vi "Scan Module.vi"(7 "Slice pattern":T1={"repitition"=14, "thick slice (um)"=500.0, "thin slice (um)"=100.0} {"thin slice (um)" format="%#_13g"; "thick slice (um)" format="%#_13g"}, 8 "Error In":errorcluster, 9 "System Parameters":T2={"Vibratome"={"Z Bottom [mm]"=0.0, "Pre Cut Dwell [s]"=1.0, "Blade Frequency [RPM]"=3000, "Slice Speed [mm/s]"=0.1, "Post Cut Dwell [s]"=4.0, "Ramp Time [s]"=0.5, "Start X [mm]"=80.5, "Start Y [mm]"=72.0, "Slice Length [mm]"=15.0, "Slice Axis"=enum."X Axis", "Controller VISA Ref"="COM3"}, "Table Stages"={"X Stage"={"Position"=0.0, "Is.Enabled?"=FALSE, "Is.Connected?"=FALSE, "Device SN"="45875688", "AccelerationMaximum"=50.0, "VelocityMaximum"=50.0, "Acceleration"=20.0, "Velocity"=20.0, "waitTimeout (ms)"=1000000, "Model"=enum."Thorlabs LTS", "Is.Homed?"=FALSE}, "Y Stage"={"Position"=0.0, "Is.Enabled?"=FALSE, "Is.Connected?"=FALSE, "Device SN"="45875512", "AccelerationMaximum"=50.0, "VelocityMaximum"=50.0, "Acceleration"=20.0, "Velocity"=20.0, "waitTimeout (ms)"=1000000, "Model"=enum."Thorlabs LTS", "Is.Homed?"=FALSE}, "Z Stage"={"Position"=0.0, "Is.Enabled?"=FALSE, "Is.Connected?"=FALSE, "Device SN"="49872414", "AccelerationMaximum"=50.0, "VelocityMaximum"=50.0, "Acceleration"=20.0, "Velocity"=20.0, "waitTimeout (ms)"=100000, "Model"=enum."Thorlabs MLJ", "Is.Homed?"=FALSE}}}, 10 "Mosaic Parameters":T5={"Overlap Options"={"Overlap Type"=enum."No Overlap", "Percent Overlap"=0, "Justify"=enum."Start"}, "Mosaic Range"={"X Axis"={"Start [mm]"=10.0, "Steps [pts]"=0, "End [mm]"=28.0}, "Y Axis"={"Start [mm]"=45.0, "Steps [pts]"=0, "End [mm]"=63.0}}, "Scan Pattern"=enum."Uni-directional", "Number of slices"=1} {"Overlap Options"."Percent Overlap" max=50}, 11 "Imaging Parameters":T6={"Save Path"=path "E:/Jiarui/1217test", "# Cscan"=1, "ROI Parameters"={"ROI (mm)"={"X (mm)"=1.0, "Y (mm)"=1.0}, "Shift (mm)"={"Xshift (mm)"=0.0, "Yshift (mm)"=0.0}}, "Scan Parameters"={"# Scan"={"#Ascan"=400, "#Bscan"=400}, "# Rpt"={"#ARpt"=1, "#BRpt"=1}, "Aline Rate"=2, "# Extra"={"# ARpt_extra"=5, "#Brtn_extra"=80}}, "Objective"=0, "Image Index"=0} {"Objective" items=["5X LKM05", "10X LKM10", "20X LKM20", "10X LSM02"]; "Scan Parameters"."Aline Rate" items=["76 KHz", "146 KHz", "76 KHz", "28 KHz", "10 KHz"]}) -> (0 "Error Out":errorcluster, 3 "Finished?":bool)   [LabVIEW 2017]
uses:
  Controls/Go Scan Actions.ctl
  Controls/System Parameters.ctl
  Hardware/Table Stage/Controls/Translation Stage Cluster.ctl
  Controls/Translation Stage Types.ctl
  Controls/FGV Actions.ctl
  Controls/ScanType.ctl
  Hardware/Table Stage/Controls/Motion Translation Module Control.ctl
  Controls/Set Get Controls.ctl
panel:
  out "Waveform Chart":dbl(graph)
  out "Current State":T7
  out "Current Position":cluster{"X":dbl, "Y":dbl}
  out "XY Graph":cluster{"X":dbl, "Y":dbl}[](graph)
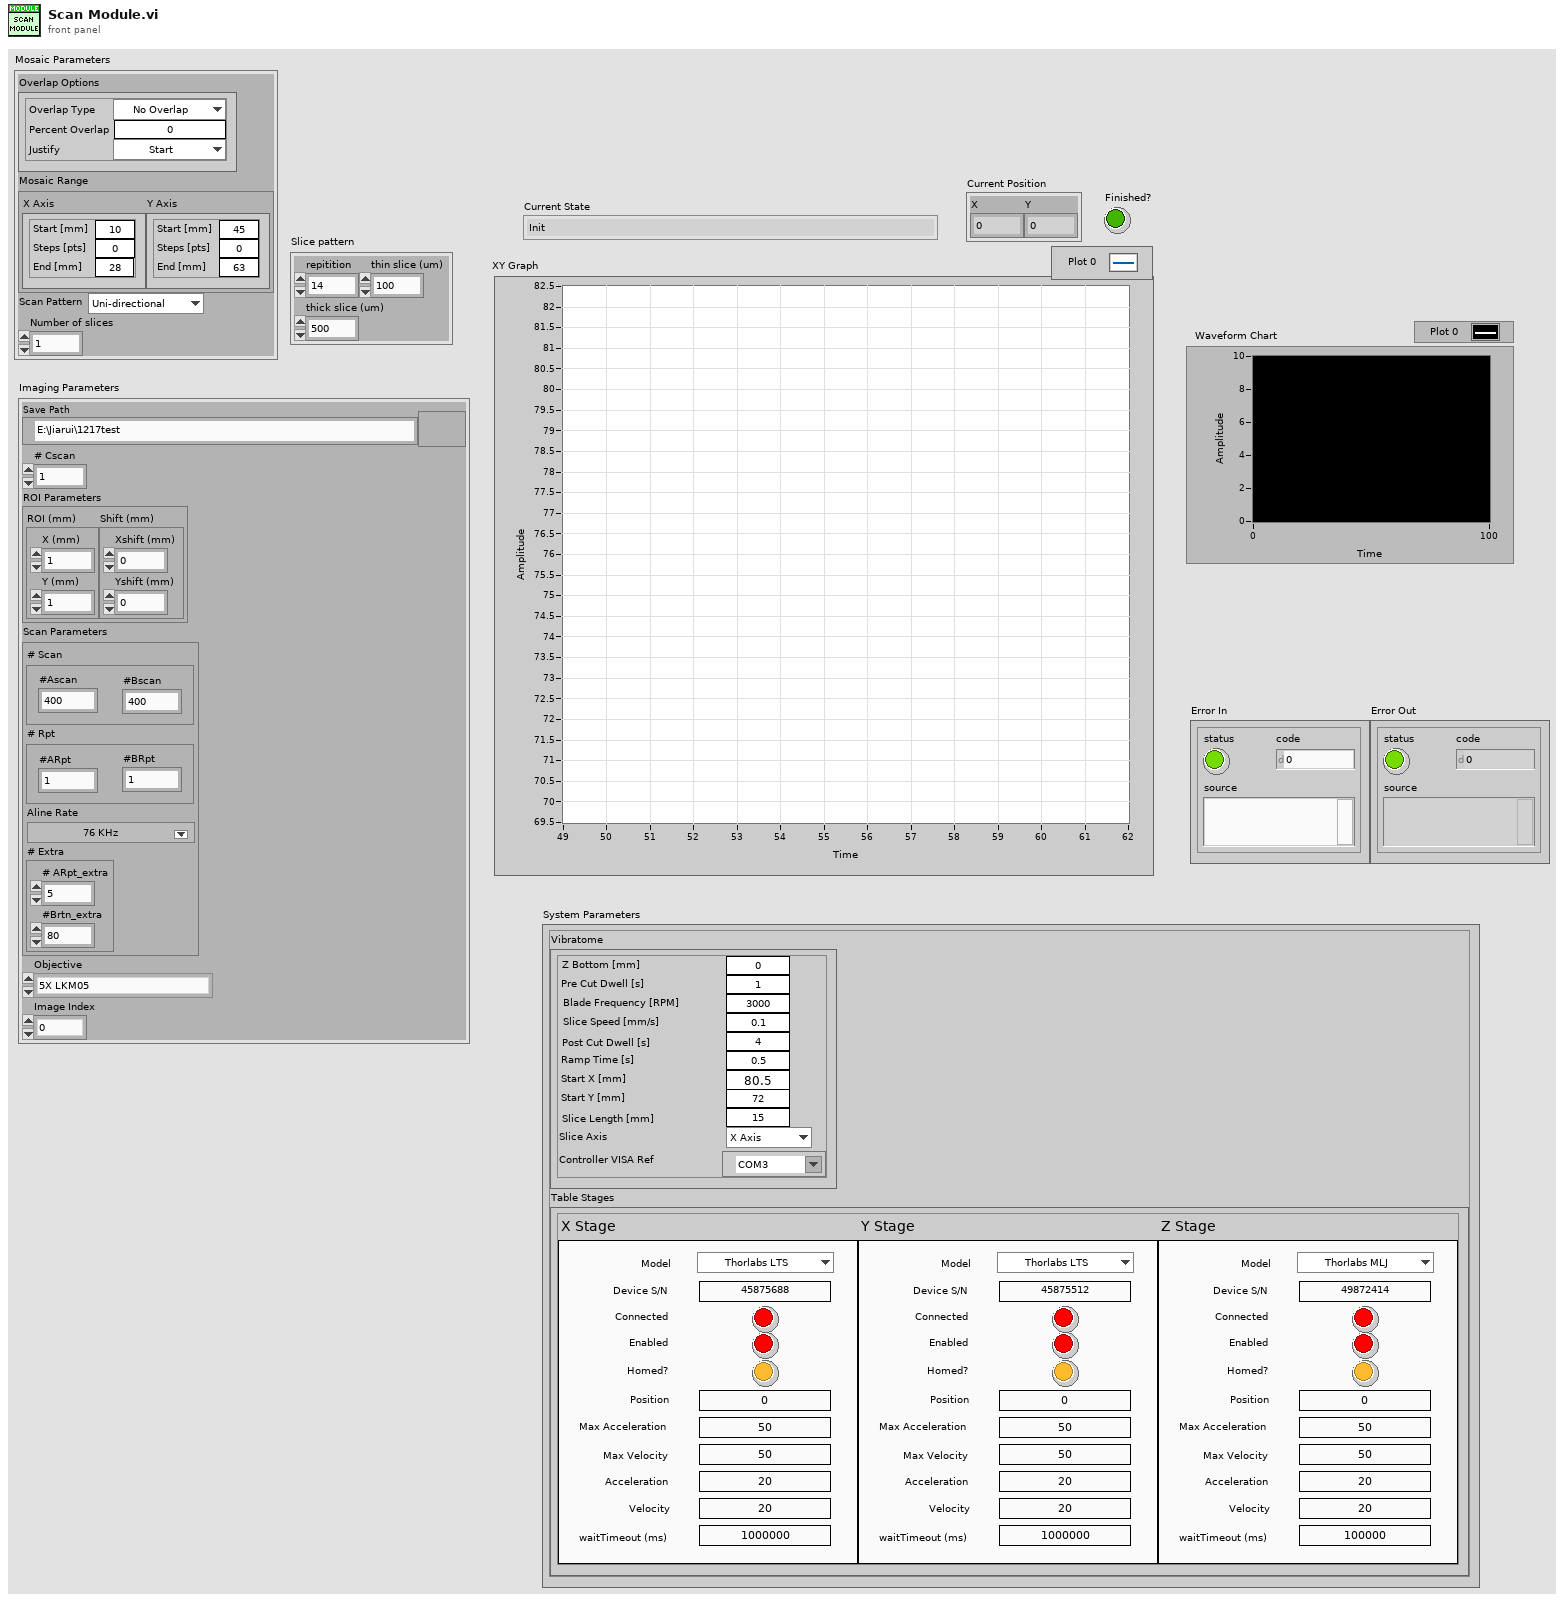
[diagram p1: front panel]
types:
  T1 = cluster{"repitition":i32, "thick slice (um)":dbl, "thin slice (um)":dbl}
  T2 = typedef "System Parameters.ctl" = cluster{"Vibratome":cluster{"Z Bottom [mm]":dbl, "Pre Cut Dwell [s]":dbl, "Blade Frequency [RPM]":u16, "Slice Speed [mm/s]":dbl, "Post Cut Dwell [s]":dbl, "Ramp Time [s]":dbl, "Start X [mm]":dbl, "Start Y [mm]":dbl, "Slice Length [mm]":dbl, "Slice Axis":enum16{"X Axis", "Y Axis", "Z Axis"}, "Controller VISA Ref":refnum<visa-resource-name>}, "Table Stages":cluster{"X Stage":T3, "Y Stage":T3, "Z Stage":T3}}
  T3 = typedef "Translation Stage Cluster.ctl" = cluster{"Position":dbl, "Is.Enabled?":bool, "Is.Connected?":bool, "Device SN":string, "AccelerationMaximum":dbl, "VelocityMaximum":dbl, "Acceleration":dbl, "Velocity":dbl, "waitTimeout (ms)":i32, "Model":T4, "Is.Homed?":bool}
  T4 = typedef "Translation Stage Types.ctl" = enum16{"None", "Thorlabs LTS", "Thorlabs MLJ"}
  T5 = cluster{"Overlap Options":cluster{"Overlap Type":enum16{"No Overlap", "X Only", "Y Only", "X and Y"}, "Percent Overlap":u8, "Justify":enum16{"Start", "Center", "End"}}, "Mosaic Range":cluster{"X Axis":cluster{"Start [mm]":dbl, "Steps [pts]":u16, "End [mm]":dbl}, "Y Axis":cluster{"Start [mm]":dbl, "Steps [pts]":u16, "End [mm]":dbl}}, "Scan Pattern":enum16{"Uni-directional", "Bi-Directional", "Spiral Out", "Spiral In"}, "Number of slices":i16}
  T6 = cluster{"Save Path":path, "# Cscan":i32, "ROI Parameters":cluster{"ROI (mm)":cluster{"X (mm)":sgl, "Y (mm)":sgl}, "Shift (mm)":cluster{"Xshift (mm)":sgl, "Yshift (mm)":sgl}}, "Scan Parameters":cluster{"# Scan":cluster{"#Ascan":i32, "#Bscan":i32}, "# Rpt":cluster{"#ARpt":i32, "#BRpt":i32}, "Aline Rate":u16, "# Extra":cluster{"# ARpt_extra":i32, "#Brtn_extra":i32}}, "Objective":u16, "Image Index":i16}
  T7 = typedef "Go Scan Actions.ctl" = enum16{"Init", "Init Scan Head", "Init Table Stage", "Init Vibratome", "Generate Mosaic", "Go Image Home", "Go Mosaic", "Acquire Image", "Go Vibratome", "Slice", "Finished"}
  T8 = cluster{"Start [mm]":dbl, "Steps [pts]":u16, "End [mm]":dbl}
  T9 = enum16{"Uni-directional", "Bi-Directional", "Spiral Out", "Spiral In"}
  T10 = cluster{"Overlap Type":enum16{"No Overlap", "X Only", "Y Only", "X and Y"}, "Percent Overlap":u8, "Justify":enum16{"Start", "Center", "End"}}
  T11 = typedef "FGV Actions.ctl" = enum16{"Init", "Set", "Get", "Clear"}
  T12 = typedef "ScanType.ctl" = enum16{"Single Frame", "Continuous Frame", "ROI Line", "Vibratome", "Mosaic", "Mosaic + Slice"}
  T13 = enum16{"Init", "Configure", "Configure Data", "Generate Scan Pattern", "Start Acquire Raw", "Start Acquire Data", "Acquire RAW", "Acquire Data", "Stop Acquire", "Uninit"}
  T14 = enum16{"Create", "Enqueue", "Dequeue", "Release"}
  T15 = typedef "Set Get Controls.ctl" = enum16{"Set", "Get"}
  T16 = typedef "Motion Translation Module Control.ctl" = enum16{"Init", "Home", "Status", "Velocity/Accel", "Position", "Jog", "Stop", "Uninit", "Enable", "Disable"}
  T17 = cluster{"Image Index":i16, "Slice Index":i16, "#Cscan":i32, "nAT per B":i32, "nA per B":i32, "Brtn_extra/2":i32}
  T18 = cluster{"Z start (pxl)":i32, "Z length (pxl)":i32}
  T19 = cluster{"# Scan":cluster{"#Ascan":i32, "#Bscan":i32}, "# Rpt":cluster{"#ARpt":i32, "#BRpt":i32}, "Aline Rate":u16, "# Extra":cluster{"# ARpt_extra":i32, "#Brtn_extra":i32}}
  T20 = cluster{"ROI (mm)":cluster{"X (mm)":sgl, "Y (mm)":sgl}, "Shift (mm)":cluster{"Xshift (mm)":sgl, "Yshift (mm)":sgl}}
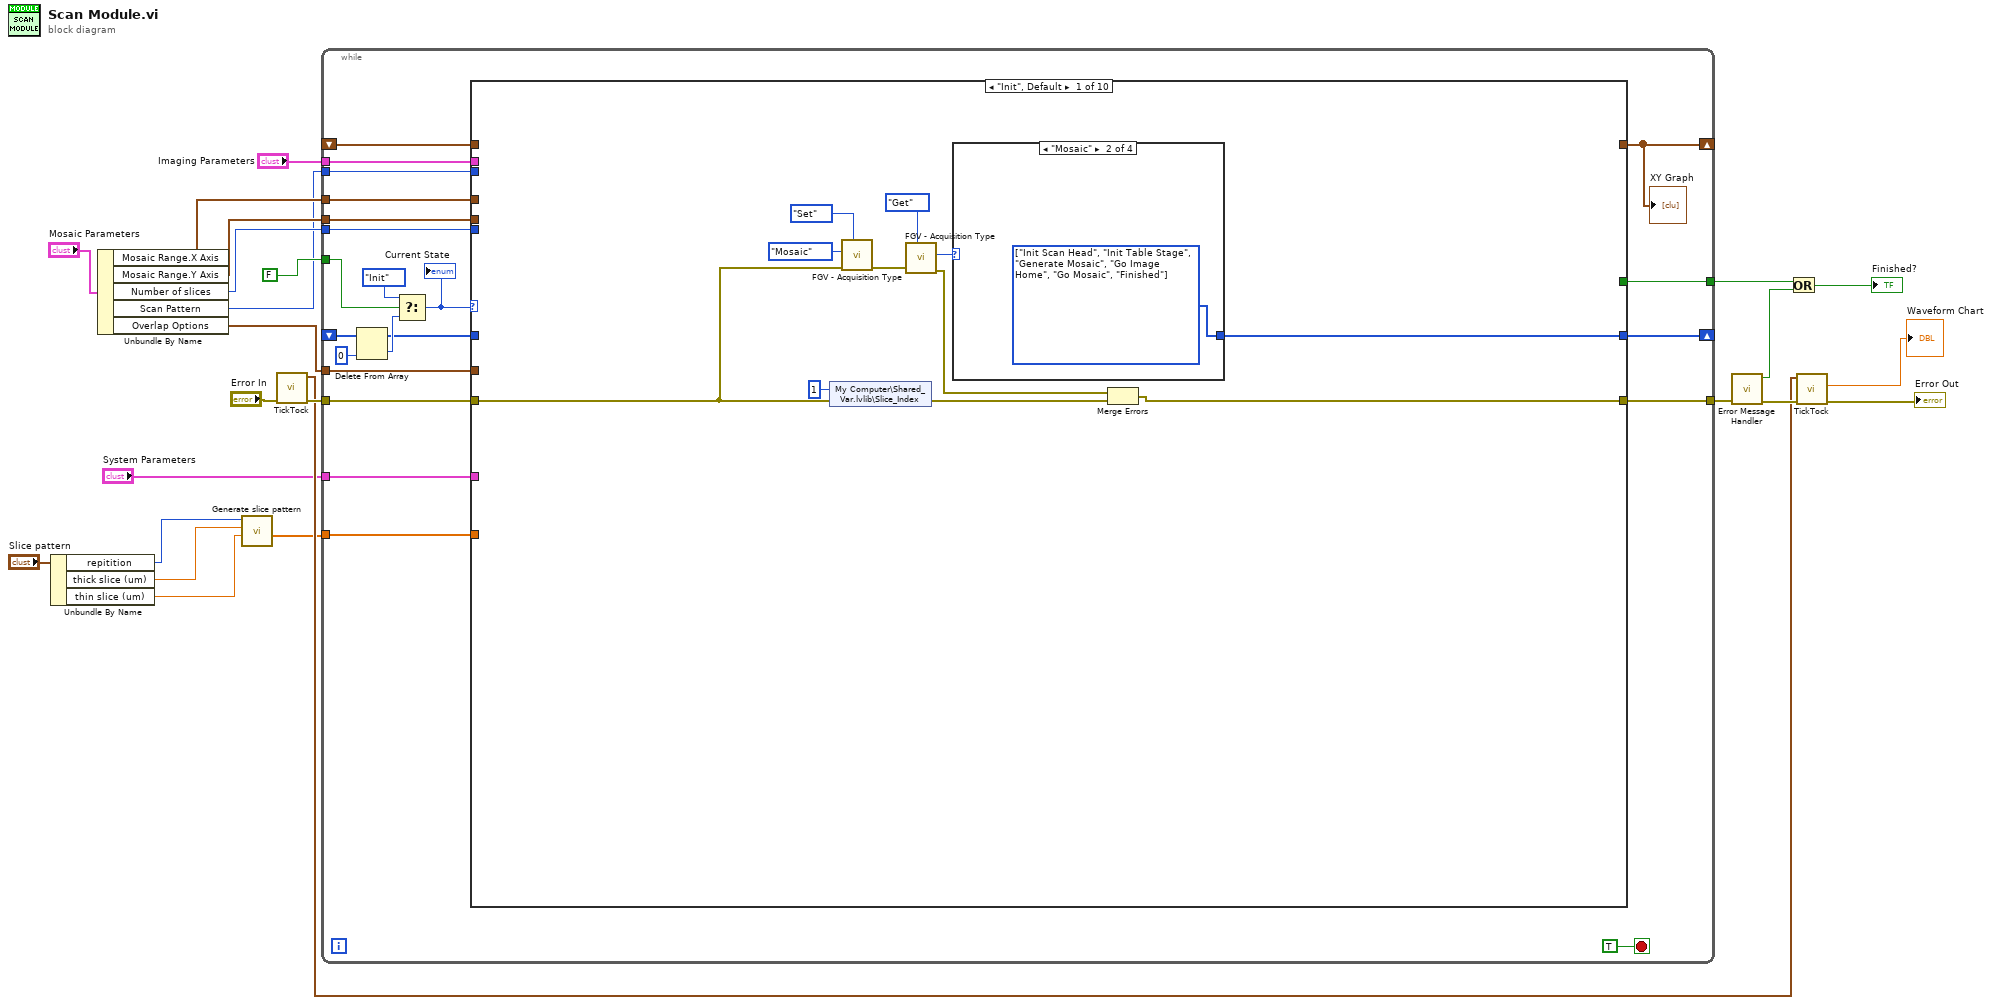
[diagram p0: block diagram]
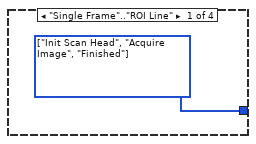
[diagram p2: hidden frame]
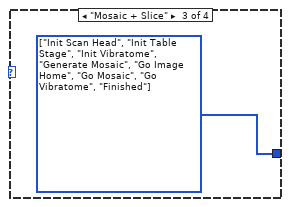
[diagram p3: hidden frame]
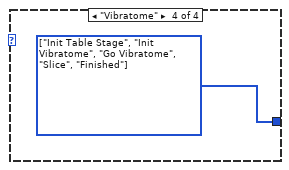
[diagram p4: hidden frame]
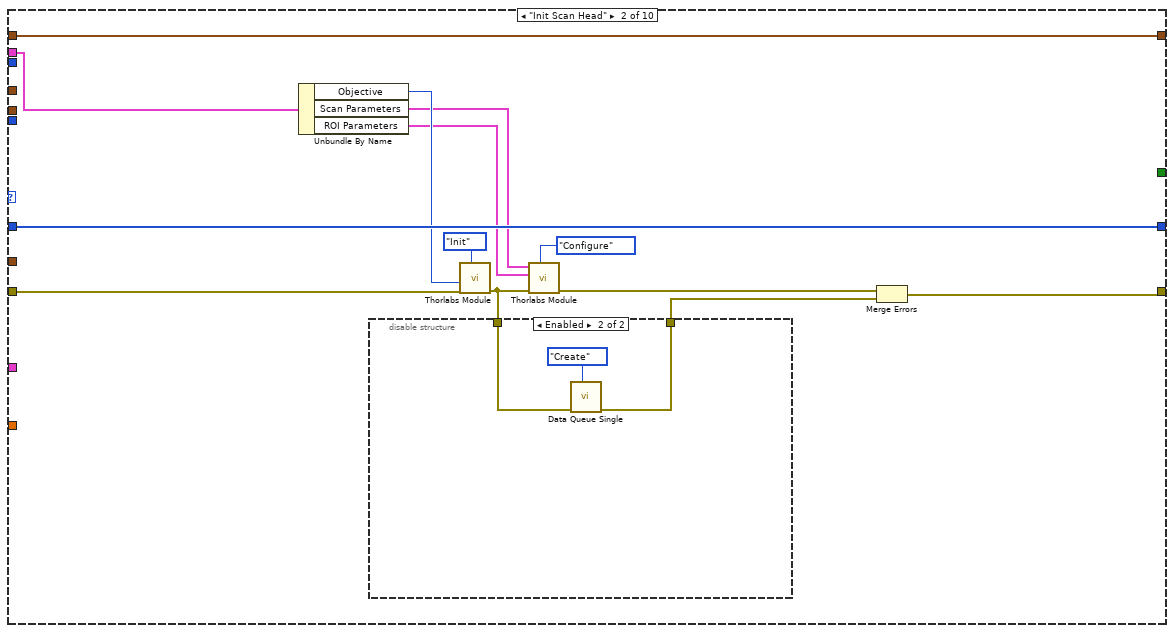
[diagram p5: hidden frame]
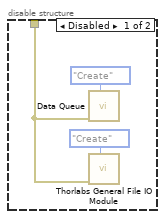
[diagram p6: hidden frame]
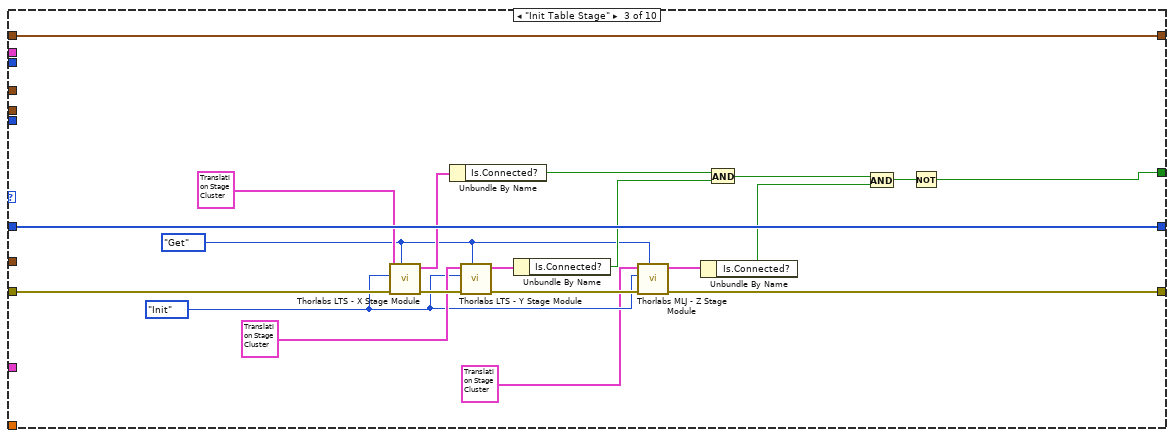
[diagram p7: hidden frame]
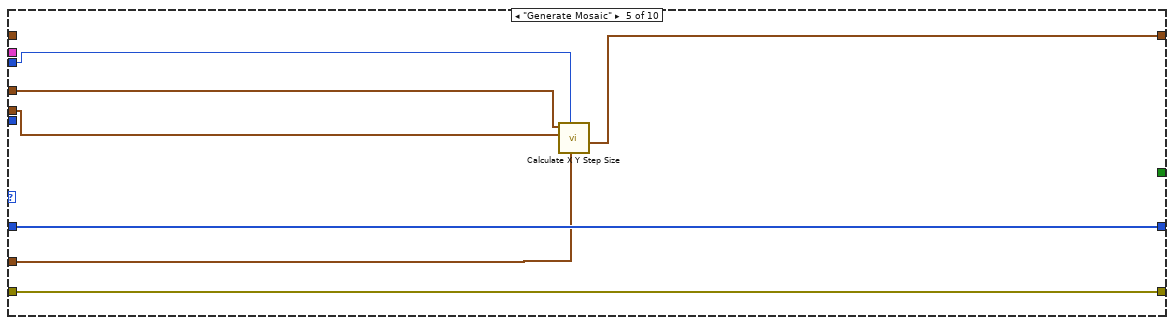
[diagram p9: hidden frame]
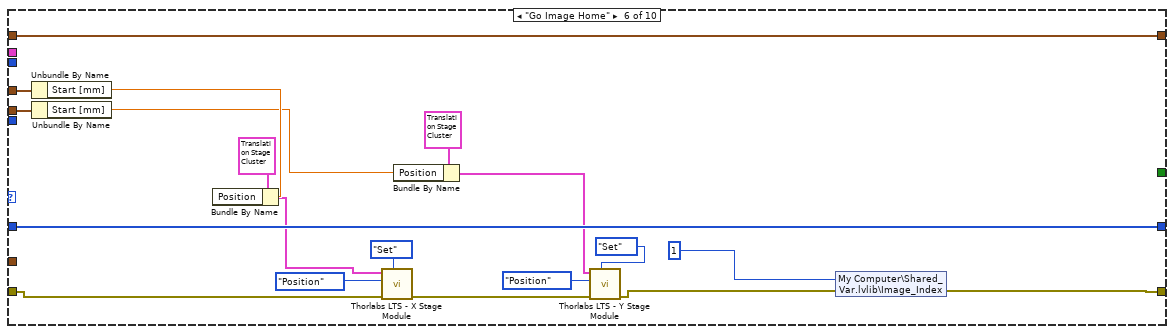
[diagram p10: hidden frame]
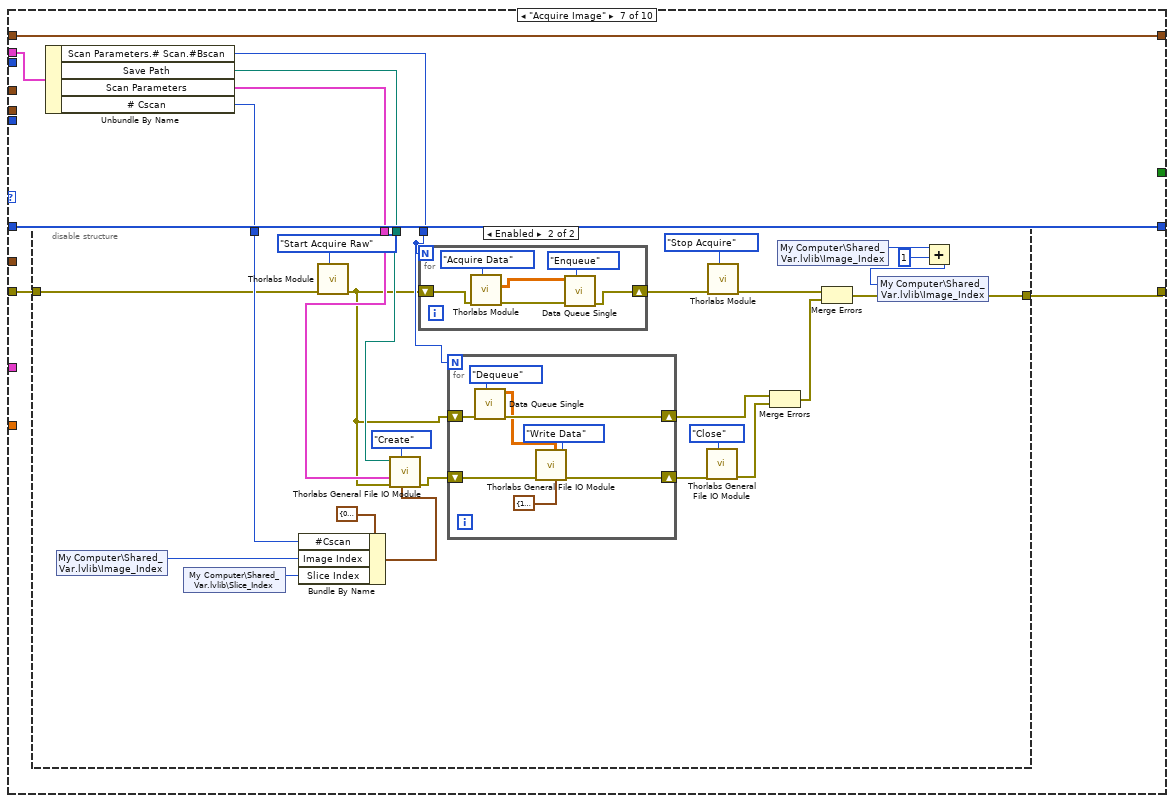
[diagram p11: hidden frame]
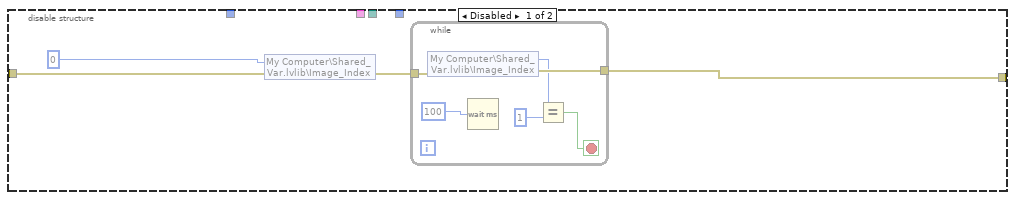
[diagram p12: hidden frame]
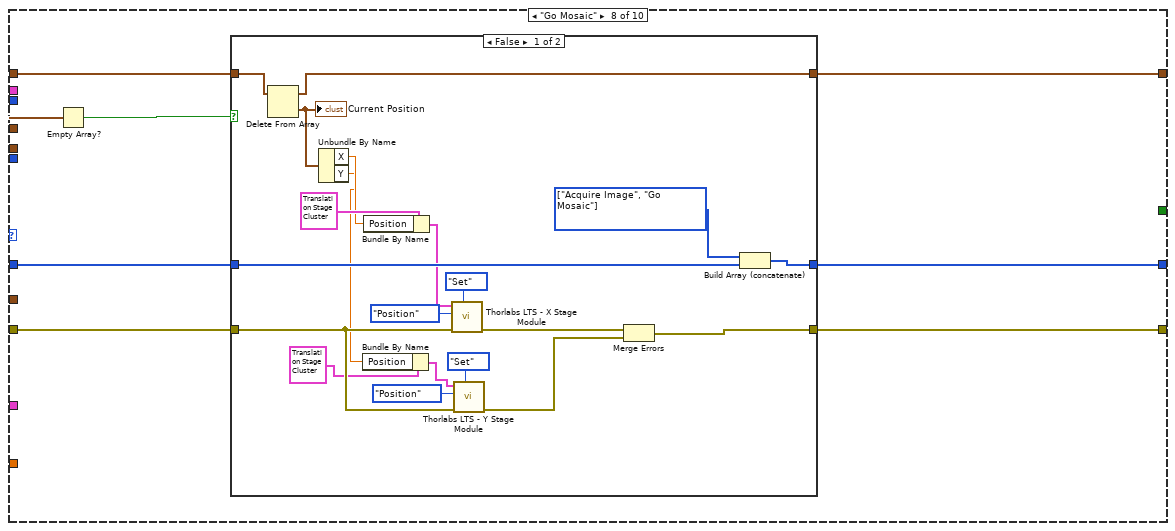
[diagram p13: hidden frame]
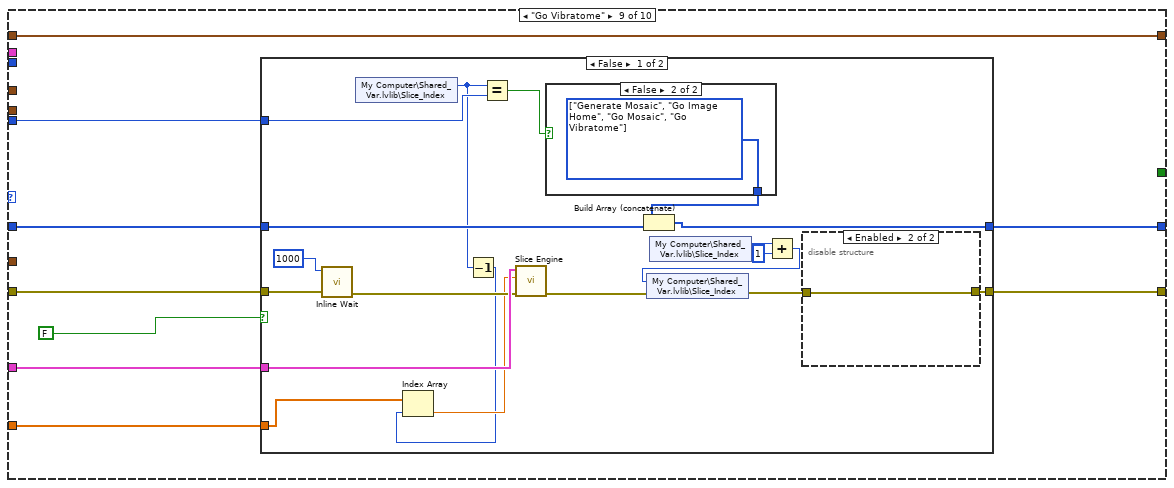
[diagram p15: hidden frame]
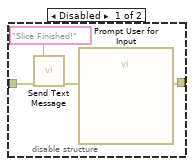
[diagram p16: hidden frame]
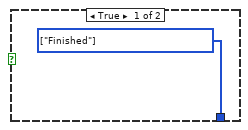
[diagram p17: hidden frame]
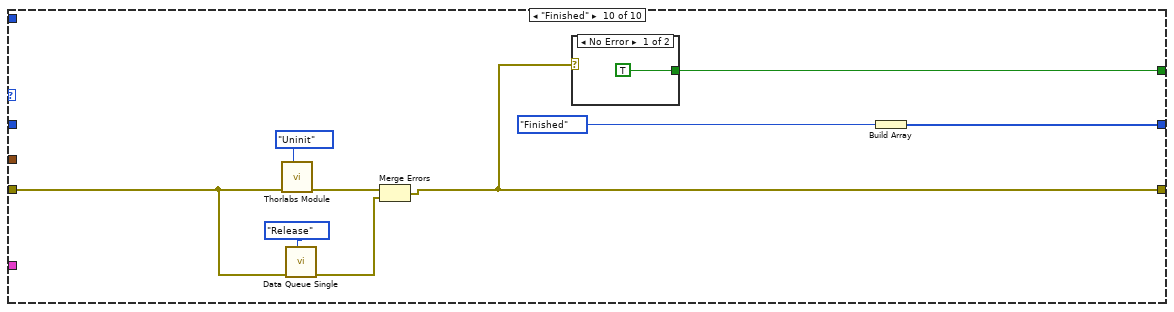
[diagram p19: hidden frame]
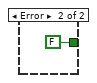
[diagram p20: hidden frame]
diagram:
  n1 = Unbundle By Name("Slice pattern") -> ("repitition"=w3:i32, "thick slice (um)"=w2:dbl, "thin slice (um)"=w1:dbl)
  n2 = Unbundle By Name("Mosaic Parameters") -> ("Mosaic Range.X Axis"=w12:T8, "Mosaic Range.Y Axis"=w11:T8, "Number of slices"=w9:i16, "Scan Pattern"=w7:T9, "Overlap Options"=w8:T10)
  n3 = call "Generate slice pattern.vi"("thin slice (um)"=w1, "thick slice (um)"=w2, "repitition"=w3) -> ("Array"=w5:dbl[])  [unwired: 8 in]
  n4 = call "TickTock.vi"("Error In"="Error In") -> ("Error Out"=w17:errorcluster, "Current Time (Out)"=w15:timestamp)  [unwired: 8 in, 1 out]
  n5 = while {
    shift-right: [w43] -> _
    shift-left: _ -> [w42]
    tunnel: FALSE ("Init") -> [w45]
    shift-right: [w38] -> _
    shift-left: _ -> [w39]
    tunnel: [w37] -> w23
    tunnel: w17 -> [w35]
    tunnel: [w34] -> w22
    tunnel: w12 -> [w32]
    tunnel: w11 -> [w31]
    tunnel: "Imaging Parameters" -> [w30]
    tunnel: w9 -> [w29]
    tunnel: w8 -> [w28]
    tunnel: w7 -> [w27]
    tunnel: "System Parameters" -> [w26]
    tunnel: w5 -> [w25]
    stop <- TRUE stop-if-true
    n6 = Delete From Array(array=w42, index=0) -> (deleted portion=w41:T7, array with subset deleted=w40:T7[])  [unwired: 1 in]
    n7 = Select(t=Go_Scan_Actions."Init", s=w45, f=w41) -> (s? t:f=w44:T7)
    "Current State" <- w44
    n8 = case shown="\"Init\", Default" w44 {
      tunnel: [w55 w73 w99 w102 w110 w128 w137 w191 w224 w263] -> w43
      tunnel: w40 -> [_ w73 w99 w102 w110 w128 w137 w192 w225 _]
      tunnel: [_ w74 w100 w103 w108 w129 w138 w195 w227 _] -> w38
      tunnel: w39 -> [_ w74 w100 w103 _ w129 w138 w194 w227 _]
      tunnel: [_ _ w94 _ _ _ _ _ _ w262] -> w37
      tunnel: w35 -> [w49 w71 w98 w101 w109 w124 w136 w190 w223 w261]
      tunnel: [w50 w64 w88 w101 w109 w127 w135 w189 w222 w256] -> w34
      tunnel: w32 -> [_ _ _ _ w107 w125 _ _ _ _]
      tunnel: w31 -> [_ _ _ _ w106 w115 _ _ _ _]
      tunnel: w30 -> [_ w72 _ _ _ _ w134 _ _ _]
      tunnel: w29 -> [_ _ _ _ _ _ _ _ w221 _]
      tunnel: w28 -> [_ _ _ _ w105 _ _ _ _ _]
      tunnel: w27 -> [_ _ _ _ w104 _ _ _ _ _]
      tunnel: w26 -> [_ _ _ _ _ _ _ _ w220 _]
      tunnel: w25 -> [_ _ _ _ _ _ _ _ w219 _]
      frame "Init", Default {
        n9 = shared-variable "My Computer\\Shared_Var.lvlib\\Slice_Index"(i16 1 ("Image_Index"), error in=w49) -> (error out=w52:errorcluster)
        n10 = call "FGV - Acquisition Type.vi"("Actions"=FGV_Actions."Set", "Error In"=w49, "Scan Type [In]"=ScanType."Mosaic") -> ("Error Out"=w53:errorcluster)  [unwired: 6 in, 2 out]
        n11 = call "FGV - Acquisition Type.vi"("Actions"=FGV_Actions."Get", "Error In"=w53) -> ("Error Out"=w51:errorcluster, "Scan Type [Out]"=w56:T12)  [unwired: 7 in, 1 out]
        n12 = case shown="\"Mosaic\"" w56 {
          tunnel: [w58 w59 w60 w61] -> w55
          frame "Single Frame".."ROI Line" {
            w58 = T7[] [enum."Init Scan Head", enum."Acquire Image", enum."Finished"] items=["Init", "Init Scan Head", "Init Table Stage", "Init Vibratome", "Generate Mosaic", "Go Image Home", "Go Mosaic", "Acquire Image", "Go Vibratome", "Slice", "Finished"]
          }
          frame "Mosaic" {
            w59 = T7[] [enum."Init Scan Head", enum."Init Table Stage", enum."Generate Mosaic", enum."Go Image Home", enum."Go Mosaic", enum."Finished"] items=["Init", "Init Scan Head", "Init Table Stage", "Init Vibratome", "Generate Mosaic", "Go Image Home", "Go Mosaic", "Acquire Image", "Go Vibratome", "Slice", "Finished"]
          }
          frame "Mosaic + Slice" {
            w60 = T7[] [enum."Init Scan Head", enum."Init Table Stage", enum."Init Vibratome", enum."Generate Mosaic", enum."Go Image Home", enum."Go Mosaic", enum."Go Vibratome", enum."Finished"] items=["Init", "Init Scan Head", "Init Table Stage", "Init Vibratome", "Generate Mosaic", "Go Image Home", "Go Mosaic", "Acquire Image", "Go Vibratome", "Slice", "Finished"]
          }
          frame "Vibratome" {
            w61 = T7[] [enum."Init Table Stage", enum."Init Vibratome", enum."Go Vibratome", enum."Slice", enum."Finished"] items=["Init", "Init Scan Head", "Init Table Stage", "Init Vibratome", "Generate Mosaic", "Go Image Home", "Go Mosaic", "Acquire Image", "Go Vibratome", "Slice", "Finished"]
          }
        }
        n13 = Merge Errors(w51, w52) -> (w50:errorcluster)
      }
      frame "Init Scan Head" {
        n14 = Unbundle By Name(w72) -> ("Objective"=w70:u16, "Scan Parameters"=w69:T19, "ROI Parameters"=w68:T20)
        n15 = call "Thorlabs Module.vi"("Actions"=T13."Init", "error in"=w71, "Objective"=w70) -> ("error out"=w67:errorcluster)  [unwired: 6 in, 2 out]
        n16 = disable-structure shown="Enabled" {
          disable-tunnel: w67 -> [w75 w79]
          disable-tunnel: [_ w78] -> w65
          frame Disabled {
            n17 = call "Data Queue.vi"("Action"=T14."Create", "error in (no error)"=w75) -> ()  [unwired: 8 in, 2 out]
            n18 = call "Thorlabs General File IO Module.vi"("Actions"=enum16{"Create", "Write", "Close"}."Create", "error in"=w75) -> ()  [unwired: 7 in, 3 out]
          }
          frame Enabled {
            n19 = call "Data Queue Single.vi"("Action"=T14."Create", "error in (no error)"=w79) -> ("error out"=w78:errorcluster)  [unwired: 8 in, 1 out]
          }
        }
        n20 = call "Thorlabs Module.vi"("Actions"=T13."Configure", "error in"=w67, "ROI Parameters"=w68, "Scan Parameters"=w69) -> ("error out"=w66:errorcluster)  [unwired: 5 in, 2 out]
        n21 = Merge Errors(w66, w65) -> (w64:errorcluster)
      }
      frame "Init Table Stage" {
        w87 = Set_Get_Controls."Get" ("Set/Get")
        w86 = Motion_Translation_Module_Control."Init" ("Action")
        n22 = call "Thorlabs LTS - X Stage Module.vi"("Set/Get"=w87, "Error In"=w98, "Action"=w86, "Cluster In"=T3 {"Position"=0.0, "Is.Enabled?"=TRUE, "Is.Connected?"=FALSE, "Device SN"="45876060", "AccelerationMaximum"=0.0, "VelocityMaximum"=0.0, "Acceleration"=0.0, "Velocity"=0.0, "waitTimeout (ms)"=10000000, "Model"=enum."Thorlabs LTS", "Is.Homed?"=FALSE}) -> ("Error Out"=w97:errorcluster, "Cluster Out"=w96:T3)  [unwired: 6 in]
        n23 = Unbundle By Name(w96) -> ("Is.Connected?"=w95:bool)
        n24 = call "Thorlabs LTS - Y Stage Module.vi"("Set/Get"=w87, "Error In"=w97, "Action"=w86, "Cluster In"=T3 {"Position"=0.0, "Is.Enabled?"=TRUE, "Is.Connected?"=FALSE, "Device SN"="45875512", "AccelerationMaximum"=0.0, "VelocityMaximum"=0.0, "Acceleration"=0.0, "Velocity"=0.0, "waitTimeout (ms)"=1000000, "Model"=enum."Thorlabs LTS", "Is.Homed?"=FALSE}) -> ("Error Out"=w89:errorcluster, "Cluster Out"=w91:T3)  [unwired: 6 in]
        n25 = Unbundle By Name(w91) -> ("Is.Connected?"=w90:bool)
        n26 = call "Thorlabs MLJ - Z Stage Module.vi"("Set/Get"=w87, "Error In"=w89, "Action"=w86, "Cluster In"=T3 {"Position"=0.0, "Is.Enabled?"=TRUE, "Is.Connected?"=FALSE, "Device SN"="49872414", "AccelerationMaximum"=0.0, "VelocityMaximum"=0.0, "Acceleration"=0.0, "Velocity"=0.0, "waitTimeout (ms)"=1000000, "Model"=enum."Thorlabs MLJ", "Is.Homed?"=FALSE}) -> ("Error Out"=w88:errorcluster, "Cluster Out"=w84:T3)  [unwired: 6 in]
        n27 = Unbundle By Name(w84) -> ("Is.Connected?"=w83:bool)
        n28 = And(x=w95, y=w90) -> (x .and. y?=w82:bool)
        n29 = And(x=w82, y=w83) -> (x .and. y?=w81:bool)
        n30 = Not(x=w81) -> (.not. x?=w94:bool)
      }
      frame "Init Vibratome" {
      }
      frame "Generate Mosaic" {
        n31 = call "Calculate X Y Step Size.vi"("Overlap Options"=w105, "Scan Pattern"=w104, "Y Axis"=w106, "X Axis"=w107) -> ("Array"=w108:cluster{"X":dbl, "Y":dbl}[])  [unwired: 4 in, 3 out]
      }
      frame "Go Image Home" {
        n32 = Unbundle By Name(w125) -> ("Start [mm]"=w120:dbl)
        n33 = Unbundle By Name(w115) -> ("Start [mm]"=w114:dbl)
        n34 = Bundle By Name(cluster=T3 {"Position"=0.0, "Is.Enabled?"=FALSE, "Is.Connected?"=FALSE, "Device SN"="45876060", "AccelerationMaximum"=0.0, "VelocityMaximum"=0.0, "Acceleration"=0.0, "Velocity"=0.0, "waitTimeout (ms)"=10000000, "Model"=enum."Thorlabs LTS", "Is.Homed?"=FALSE} ("Cluster In"), "Position"=w120) -> (w119:T3)
        n35 = call "Thorlabs LTS - X Stage Module.vi"("Set/Get"=Set_Get_Controls."Set", "Error In"=w124, "Action"=Motion_Translation_Module_Control."Position", "Cluster In"=w119) -> ("Error Out"=w113:errorcluster)  [unwired: 6 in, 1 out]
        n36 = Bundle By Name(cluster=T3 {"Position"=0.0, "Is.Enabled?"=FALSE, "Is.Connected?"=FALSE, "Device SN"="45875512", "AccelerationMaximum"=0.0, "VelocityMaximum"=0.0, "Acceleration"=0.0, "Velocity"=0.0, "waitTimeout (ms)"=10000000, "Model"=enum."Thorlabs LTS", "Is.Homed?"=FALSE} ("Cluster In"), "Position"=w114) -> (w118:T3)
        n37 = call "Thorlabs LTS - Y Stage Module.vi"("Set/Get"=Set_Get_Controls."Set", "Error In"=w113, "Action"=Motion_Translation_Module_Control."Position", "Cluster In"=w118) -> ("Error Out"=w112:errorcluster)  [unwired: 6 in, 1 out]
        n38 = shared-variable "My Computer\\Shared_Var.lvlib\\Image_Index"(i16 1 ("Image_Index"), error in=w112) -> (error out=w127:errorcluster)
      }
      frame "Acquire Image" {
        n39 = Unbundle By Name(w134) -> ("Scan Parameters.# Scan.#Bscan"=w133:i32, "Save Path"=w132:path, "Scan Parameters"=w131:T19, "# Cscan"=w130:i32)
        n40 = disable-structure shown="Enabled" {
          disable-tunnel: w136 -> [w141 w149]
          disable-tunnel: [w139 w166] -> w135
          disable-tunnel: w133 -> [_ w170]
          disable-tunnel: w132 -> [_ w158]
          disable-tunnel: w131 -> [_ w156]
          disable-tunnel: w130 -> [_ w171]
          frame Disabled {
            n41 = shared-variable "My Computer\\Shared_Var.lvlib\\Image_Index"(i16 0 ("Image_Status"), error in=w141) -> (error out=w140:errorcluster)
            n42 = while {
              tunnel: w140 -> [w147]
              tunnel: [w146] -> w139
              stop <- w145 stop-if-true
              n43 = shared-variable "My Computer\\Shared_Var.lvlib\\Image_Index"(error in=w147) -> (w144:i16, error out=w146:errorcluster)
              n44 = Wait (ms)(milliseconds to wait=u32 100) -> ()  [unwired: 1 out]
              n45 = Equal?(x=w144, y=i16 1) -> (x = y?=w145:bool)
            }
          }
          frame Enabled {
            n46 = shared-variable "My Computer\\Shared_Var.lvlib\\Image_Index"() -> (w160:i16)  [unwired: 1 in, 1 out]
            n47 = shared-variable "My Computer\\Shared_Var.lvlib\\Slice_Index"() -> (w162:i16)  [unwired: 1 in, 1 out]
            n48 = Bundle By Name(cluster=T17 {"Image Index"=0, "Slice Index"=0, "#Cscan"=0, "nAT per B"=0, "nA per B"=0, "Brtn_extra/2"=0} ("input cluster"), "#Cscan"=w171, "Image Index"=w160, "Slice Index"=w162) -> (w157:T17)
            n49 = call "Thorlabs Module.vi"("Actions"=T13."Start Acquire Raw", "error in"=w149) -> ("error out"=w155:errorcluster)  [unwired: 7 in, 2 out]
            n50 = call "Thorlabs General File IO Module.vi"("Imaging Parameters"=w157, "Actions"=enum16{"Create", "Write", "Write Data", "Close"}."Create", "error in"=w155, "Scan Parameters"=w156, "Save Path"=w158) -> ("error out"=w159:errorcluster)  [unwired: 4 in, 2 out]
            n51 = for {
              N: w170 -> [_]
              shift-right: [w185] -> w173
              shift-left: w155 -> [w188]
              n52 = call "Thorlabs Module.vi"("Actions"=T13."Acquire Data", "error in"=w188) -> ("error out"=w186:errorcluster, "Data Out"=w183:sgl[][])  [unwired: 7 in, 1 out]
              n53 = call "Data Queue Single.vi"("Action"=T14."Enqueue", "error in (no error)"=w186, "Data In"=w183) -> ("error out"=w185:errorcluster)  [unwired: 7 in, 1 out]
            }
            n54 = for {
              N: w170 -> [_]
              shift-right: [w181] -> w154
              shift-left: w155 -> [w180]
              shift-right: [w179] -> w163
              shift-left: w159 -> [w178]
              n55 = call "Data Queue Single.vi"("Action"=T14."Dequeue", "error in (no error)"=w180) -> ("error out"=w181:errorcluster, "Data Out"=w176:sgl[][])  [unwired: 8 in]
              n56 = call "Thorlabs General File IO Module.vi"("Data Range"=T18 {"Z start (pxl)"=1, "Z length (pxl)"=400}, "Data In"=w176, "Actions"=enum16{"Create", "Write", "Write Data", "Close"}."Write Data", "error in"=w178) -> ("error out"=w179:errorcluster)  [unwired: 5 in, 2 out]
            }
            n57 = call "Thorlabs General File IO Module.vi"("Actions"=enum16{"Create", "Write", "Write Data", "Close"}."Close", "error in"=w163) -> ("error out"=w164:errorcluster)  [unwired: 7 in, 2 out]
            n58 = call "Thorlabs Module.vi"("Actions"=T13."Stop Acquire", "error in"=w173) -> ("error out"=w172:errorcluster)  [unwired: 7 in, 2 out]
            n59 = Merge Errors(w154, w164) -> (w174:errorcluster)
            n60 = shared-variable "My Computer\\Shared_Var.lvlib\\Image_Index"() -> (w169:i16)  [unwired: 1 in, 1 out]
            n61 = Merge Errors(w172, w174) -> (w167:errorcluster)
            n62 = Add(x=w169, y=i16 1) -> (x+y=w165:i16)
            n63 = shared-variable "My Computer\\Shared_Var.lvlib\\Image_Index"(w165, error in=w167) -> (error out=w166:errorcluster)
          }
        }
      }
      frame "Go Mosaic" {
        n64 = Empty Array?(array=w194) -> (empty?=w193:bool)
        n65 = case shown="False" w193 {
          tunnel: [w215 w218] -> w195
          tunnel: w194 -> [w214 w218]
          tunnel: w192 -> [w213 w217]
          tunnel: [w211 w217] -> w191
          tunnel: w190 -> [w201 w216]
          tunnel: [w197 w216] -> w189
          frame False {
            w210 = T7[] [enum."Acquire Image", enum."Go Mosaic"] items=["Init", "Init Scan Head", "Init Table Stage", "Init Vibratome", "Generate Mosaic", "Go Image Home", "Go Mosaic", "Acquire Image", "Go Vibratome", "Slice", "Finished"]
            n66 = Delete From Array(array=w214) -> (deleted portion=w212:cluster{"X":dbl, "Y":dbl}, array with subset deleted=w215:cluster{"X":dbl, "Y":dbl}[])  [unwired: 2 in]
            "Current Position" <- w212
            n67 = Unbundle By Name(w212) -> ("X"=w205:dbl, "Y"=w199:dbl)
            n68 = Bundle By Name(cluster=T3 {"Position"=0.0, "Is.Enabled?"=FALSE, "Is.Connected?"=FALSE, "Device SN"="45875512", "AccelerationMaximum"=0.0, "VelocityMaximum"=0.0, "Acceleration"=0.0, "Velocity"=0.0, "waitTimeout (ms)"=10000000, "Model"=enum."None", "Is.Homed?"=FALSE} ("Cluster In"), "Position"=w199) -> (w198:T3)
            n69 = Bundle By Name(cluster=T3 {"Position"=0.0, "Is.Enabled?"=FALSE, "Is.Connected?"=FALSE, "Device SN"="45875688", "AccelerationMaximum"=0.0, "VelocityMaximum"=0.0, "Acceleration"=0.0, "Velocity"=0.0, "waitTimeout (ms)"=10000000, "Model"=enum."None", "Is.Homed?"=FALSE} ("Cluster In"), "Position"=w205) -> (w204:T3)
            n70 = call "Thorlabs LTS - X Stage Module.vi"("Set/Get"=Set_Get_Controls."Set", "Error In"=w201, "Action"=Motion_Translation_Module_Control."Position", "Cluster In"=w204) -> ("Error Out"=w208:errorcluster)  [unwired: 6 in, 1 out]
            n71 = call "Thorlabs LTS - Y Stage Module.vi"("Set/Get"=Set_Get_Controls."Set", "Error In"=w201, "Action"=Motion_Translation_Module_Control."Position", "Cluster In"=w198) -> ("Error Out"=w196:errorcluster)  [unwired: 6 in, 1 out]
            n72 = Merge Errors(w208, w196) -> (w197:errorcluster)
            n73 = Build Array (concatenate)(w210, w213) -> (w211:T7[])
          }
          frame True {
          }
        }
      }
      frame "Go Vibratome" {
        n74 = case shown="False" FALSE ("No Slice?") {
          tunnel: w225 -> [w246 w255]
          tunnel: [w245 w255] -> w224
          tunnel: w223 -> [w239 w254]
          tunnel: [w232 w254] -> w222
          tunnel: w221 -> [w237 _]
          tunnel: w220 -> [w235 _]
          tunnel: w219 -> [w230 _]
          frame False {
            n75 = call "Inline Wait.vi"("Error In"=w239, "milliseconds to wait"=u32 1000) -> ("Error Out"=w234:errorcluster)  [unwired: 9 in]
            n76 = shared-variable "My Computer\\Shared_Var.lvlib\\Slice_Index"() -> (w229:i16)  [unwired: 1 in, 1 out]
            n77 = Decrement(x=w229) -> (x-1=w228:i16)
            n78 = Index Array(array=w230, index=w228) -> (element=w231:dbl)
            n79 = Equal?(x=w229, y=w237) -> (x = y?=w240:bool)
            n80 = call "Slice Engine.vi"("error in (no error)"=w234, "Slice thickness  (mm)"=w231, "System Parameters"=w235) -> ("error out"=w236:errorcluster)  [unwired: 8 in]
            n81 = case shown="False" w240 {
              tunnel: [w252 w253] -> w244
              frame True {
                w252 = T7[] [enum."Finished"] items=["Init", "Init Scan Head", "Init Table Stage", "Init Vibratome", "Generate Mosaic", "Go Image Home", "Go Mosaic", "Acquire Image", "Go Vibratome", "Slice", "Finished"]
              }
              frame False {
                w253 = T7[] [enum."Generate Mosaic", enum."Go Image Home", enum."Go Mosaic", enum."Go Vibratome"] items=["Init", "Init Scan Head", "Init Table Stage", "Init Vibratome", "Generate Mosaic", "Go Image Home", "Go Mosaic", "Acquire Image", "Go Vibratome", "Slice", "Finished"]
              }
            }
            n82 = Build Array (concatenate)(w244, w246) -> (w245:T7[])
            n83 = shared-variable "My Computer\\Shared_Var.lvlib\\Slice_Index"() -> (w243:i16)  [unwired: 1 in, 1 out]
            n84 = Add(x=w243, y=i16 1) -> (x+y=w241:i16)
            n85 = shared-variable "My Computer\\Shared_Var.lvlib\\Slice_Index"(w241, error in=w236) -> (error out=w233:errorcluster)
            n86 = disable-structure shown="Enabled" {
              disable-tunnel: w233 -> [w250 w251]
              disable-tunnel: [w249 w251] -> w232
              frame Disabled {
                n87 = call "Send Text Message.vi"("error in"=w250, "subject"="Slice Finished!") -> ("error out"=w248:errorcluster)  [unwired: 9 in]
                n88 = call "Prompt User for Input"("error in (no error)"=w248) -> ("error out"=w249:errorcluster)  [unwired: 17 in, 1 out]
              }
              frame Enabled {
              }
            }
          }
          frame True {
          }
        }
      }
      frame "Finished" {
        n89 = call "Thorlabs Module.vi"("Actions"=T13."Uninit", "error in"=w261) -> ("error out"=w259:errorcluster)  [unwired: 7 in, 2 out]
        n90 = call "Data Queue Single.vi"("Action"=T14."Release", "error in (no error)"=w261) -> ("error out"=w258:errorcluster)  [unwired: 8 in, 1 out]
        n91 = Merge Errors(w259, w258) -> (w256:errorcluster)
        n92 = case shown="No Error" w256 {
          tunnel: [TRUE FALSE] -> w262
          frame No Error {
          }
          frame Error {
          }
        }
        n93 = Build Array(Go_Scan_Actions."Finished") -> (w263:T7[])
      }
    }
    "XY Graph" <- w38
  }
  n94 = call "Error Message Handler.vi"("Error In"=w22) -> ("Error Out"=w21:errorcluster, "T button?"=w19:bool)  [unwired: 9 in]
  n95 = Or(x=w23, y=w19) -> (x .or. y?=→"Finished?":bool)
  n96 = call "TickTock.vi"("Error In"=w21, "Current Time (In)"=w15) -> ("Error Out"=→"Error Out":errorcluster, "dt"=→"Waveform Chart":dbl)  [unwired: 7 in, 1 out]
